vi "change color.vi"(4 "Sensor 5":fxp<+,32,8>, 5 "Sensor 8":fxp<+,64,16>, 6 "Sensor 6":fxp<+,64,16>, 7 "Sensor 7":fxp<+,64,16>, 8 "Slide Refnum 4":refnum<vi>, 9 "Slide Refnum 3":refnum<vi>, 10 "Slide Refnum in":refnum<vi>, 11 "Slide in":refnum<vi>) -> (0 "Sensor 3":dbl(slide) scale=0.0..30.0, 1 "Sensor 4":dbl(slide) scale=0.0..30.0, 2 "Sensor 1":dbl(slide) scale=0.0..30.0, 3 "Sensor 2":dbl(slide) scale=0.0..30.0)   [LabVIEW 2014]
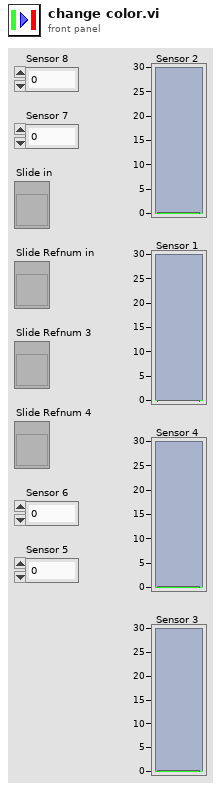
[diagram p1: front panel]
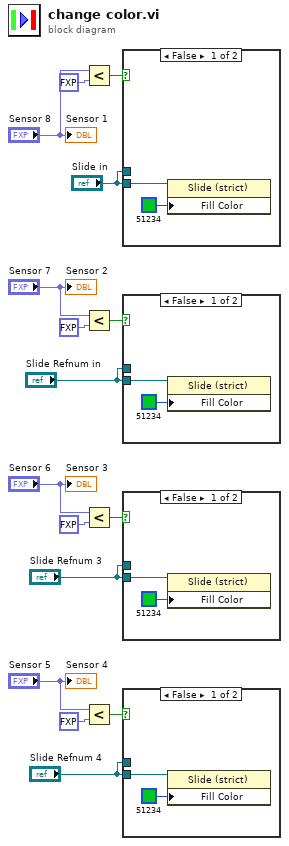
[diagram p0: block diagram]
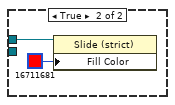
[diagram p2: hidden frame]
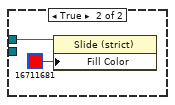
[diagram p3: hidden frame]
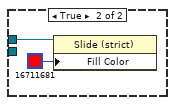
[diagram p4: hidden frame]
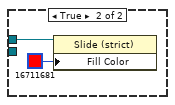
[diagram p5: hidden frame]
diagram:
  n1 = Less?(x="Sensor 8", y=fxp<+,64,16> 5.0) -> (x < y?=w7:bool)
  n2 = Less?(x="Sensor 7", y=fxp<+,64,16> 5.0) -> (x < y?=w14:bool)
  n3 = Less?(x="Sensor 6", y=fxp<+,64,16> 5.0) -> (x < y?=w15:bool)
  n4 = Less?(x="Sensor 5", y=fxp<+,64,16> 5.0) -> (x < y?=w16:bool)
  n5 = case shown="False" w7 {
    tunnel: "Slide in" -> [w17 _]
    tunnel: "Slide in" -> [_ w19]
    frame False {
      n6 = property on="Property Node" class="Slide (strict)"(reference=w17, "Fill Color"=u32 51234) -> ()  [unwired: 1 in, 2 out]
    }
    frame True {
      n7 = property on="Property Node" class="Slide (strict)"(reference=w19, "Fill Color"=u32 16711681) -> ()  [unwired: 1 in, 2 out]
    }
  }
  n8 = case shown="False" w14 {
    tunnel: "Slide Refnum in" -> [w21 _]
    tunnel: "Slide Refnum in" -> [_ w23]
    frame False {
      n9 = property on="Property Node" class="Slide (strict)"(reference=w21, "Fill Color"=u32 51234) -> ()  [unwired: 1 in, 2 out]
    }
    frame True {
      n10 = property on="Property Node" class="Slide (strict)"(reference=w23, "Fill Color"=u32 16711681) -> ()  [unwired: 1 in, 2 out]
    }
  }
  n11 = case shown="False" w15 {
    tunnel: "Slide Refnum 3" -> [w25 _]
    tunnel: "Slide Refnum 3" -> [_ w27]
    frame False {
      n12 = property on="Property Node" class="Slide (strict)"(reference=w25, "Fill Color"=u32 51234) -> ()  [unwired: 1 in, 2 out]
    }
    frame True {
      n13 = property on="Property Node" class="Slide (strict)"(reference=w27, "Fill Color"=u32 16711681) -> ()  [unwired: 1 in, 2 out]
    }
  }
  n14 = case shown="False" w16 {
    tunnel: "Slide Refnum 4" -> [w29 _]
    tunnel: "Slide Refnum 4" -> [_ w31]
    frame False {
      n15 = property on="Property Node" class="Slide (strict)"(reference=w29, "Fill Color"=u32 51234) -> ()  [unwired: 1 in, 2 out]
    }
    frame True {
      n16 = property on="Property Node" class="Slide (strict)"(reference=w31, "Fill Color"=u32 16711681) -> ()  [unwired: 1 in, 2 out]
    }
  }
  "Sensor 1" <- "Sensor 8"
  "Sensor 2" <- "Sensor 7"
  "Sensor 3" <- "Sensor 6"
  "Sensor 4" <- "Sensor 5"
